vi "VR Example.vi"() -> ()   [LabVIEW 2011]
uses:
  <vilib>/Platform/TimedLoop/XDataNode/timing_clust.ctl
  <vilib>/Platform/TimedLoop/XDataNode/nitl_modes.ctl
  <vilib>/Platform/TimedLoop/XDataNode/wakeup.ctl
  <vilib>/rvi/DataTransferAndStorage/Container/Common/niFpgaContainerState.ctl
  <vilib>/rvi/DataTransferAndStorage/Container/Common/niFpgaDataTypeControl.ctl
  <vilib>/rvi/DataTransferAndStorage/Container/Common/niFpgaContainerImplementationControl.ctl
  <vilib>/rvi/DataTransferAndStorage/Container/Common/niFpgaContainerArbitrationOptionsControl.ctl
  <vilib>/rvi/DataTransferAndStorage/Container/Common/niFpgaTransferTypeControl.ctl
  <vilib>/rvi/DataTransferAndStorage/Container/Common/niFpgaContainerInitializationParameters.ctl
  <vilib>/rvi/Memory/Memory_Types/niFpgaMemoryInterfaceConfiguration.ctl
  <vilib>/rvi/FIFO/Fifo_Types/niFpgaFifoControlLogicControl.ctl
  <vilib>/rvi/DataTransferAndStorage/Container/Common/niFpgaContainerMetaDataKey.ctl
  <userlib>/AES/FPGA/FPGA TypeDefs/aes_FullyCustomTeeth ActionEngine Enum.ctl
  <userlib>/_NI VeriStand FPGA Support/NI VeriStand RIO Library/Custom Device Components/Engine Simulation/Engine Simulation Globals.vi
  <userlib>/AES/FPGA/FPGA VIs/AES ECU Event Measurement - All Measurements.vi
  <vilib>/rvi/DataTransferAndStorage/Container/Common/niFpgaContainerGetUniqueNameForEmu.vi
  <vilib>/rvi/DataTransferAndStorage/Container/Common/niFpgaContainerSetEmuInfo.vi
  <vilib>/rvi/eio/common/nirviEmuReportErrorAndStop.vi
  <vilib>/rvi/Memory/Memory_Emulation/niFpgaMemoryEmulationValidateCache.vi
  <vilib>/rvi/Memory/Memory_Emulation/nirvimemoryEmulationManagerCache_InsertValue.vi
  <vilib>/Utility/error.llb/Clear Errors.vi
  <vilib>/rvi/Memory/Memory_Emulation/nirvimemoryEmulationManagerCache_GetValue.vi
  <vilib>/rvi/Memory/Memory_Emulation/nirvimemoryEmulationManagerCache_SetValue.vi
  <vilib>/rvi/DataTransferAndStorage/Container/Common/niFpgaContainerExecOnDevCompGetState.vi
  <vilib>/rvi/eio/common/nirviEmuTemplateMethod_errors.vi
  <vilib>/rvi/FIFO/Fifo_Resource/nirvififoEmulationSetSize.vi
  <vilib>/Platform/TimedLoop/XDataNode/XDataNode.xnode
  <vilib>/eio/EIONode/EIONode.xnode
  <vilib>/rvi/LocalResourceManager/LocalResourceManager.xnode
  <vilib>/rvi/DataTransferAndStorage/Container/XNode/niFpgaContainer.xnode
  <vilib>/rvi/Memory/Memory_Emulation/nirvimemoryEmulation.vi
  <vilib>/rvi/Memory/Memory_Emulation/niFpgaMemoryEmulationRefIn.vi
  <vilib>/rvi/FIFO/Fifo_Resource/nirvififoEmulationRead.vi
  <vilib>/rvi/FIFO/Fifo_Resource/nirvififoEmulationWrite.vi
  <userlib>/AES/FPGA/AES FPGA.lvlib
  <vilib>/Platform/TimedLoop/XDataNode/XDNodeRunTimeDep.lvlib
panel:
  in  "FullyCustomTeeth.Cams.Cam1.CycleAngle":bool
  in  "DataReplay.Offset.Crankshaft.CKS.1":u64
  in  "DataReplay.ReverseNegate?.Crankshaft.CKS.1":bool
  out "ECUEvent.IC 1.End Angle":u64
  out "ECUEvent.IC 1.Time Duration":u32
  out "ECUEvent.IC 1.Start Angle":u64
  out "ECUEvent.IC 1.Angle Duration":u64
  out "ECUEvent.FI 1.End Angle":u64
  out "ECUEvent.FI 1.Time Duration":u32
  out "ECUEvent.FI 1.Start Angle":u64
  out "ECUEvent.FI 1.Angle Duration":u64
  in  "FullyCustomTeeth.Cams.Cam1.First Rising?":bool
  in  "FullyCustomTeeth.Cams.Num Angles":u8=2
  in  "FullyCustomTeeth.Cams.Cam1.Offset":u64
  in  "FullyCustomTeeth.Cams.Num Profiles":u8=1
  in  "FullyCustomTeeth.Cams.Data":u64
  in  "FullyCustomTeeth.Cams.Toggle":bool
  in  "DataReplay.LoadOffset":u16
  in  "DataReplay.CycleAngle?.Crankshaft.CKS.1":bool
  in  "DataReplay.RPMThreshold.Crankshaft.CKS.1":u64
  in  "DataReplay.VScaleSlope.Crankshaft.CKS.1":u32
  in  "DataReplay.AngleToAddress.Crankshaft.CKS.1":u32
  in  "DataReplay.VScaleIntercept.Crankshaft.CKS.1":i32
  in  "DataReplay.UpdateRate.Crankshaft":u32=400
  in  "APU.Degrees per Tick":u64
  out "APU.Crank Angle":u64
  out "APU.Cycle Angle":u64
  in  "APU.Reset":bool
  in  "APU.Increment Rate":u64
  in  "DataReplay.Data":i16[](array[numeric])=[0, 0, 0, 0, 0, 0, 0, 0, 0, 0, 0, 0, 0, 0, 0, 0, 0, 0, 0, 0, 0, 0, 0, 0, 0, 0, 0, 0, 0, 0, 0, 0]
  in  "DataReplay.LoadDone":bool
  in  "DataReplay.Select":i8
  in  "DataReplay.Toggle":bool
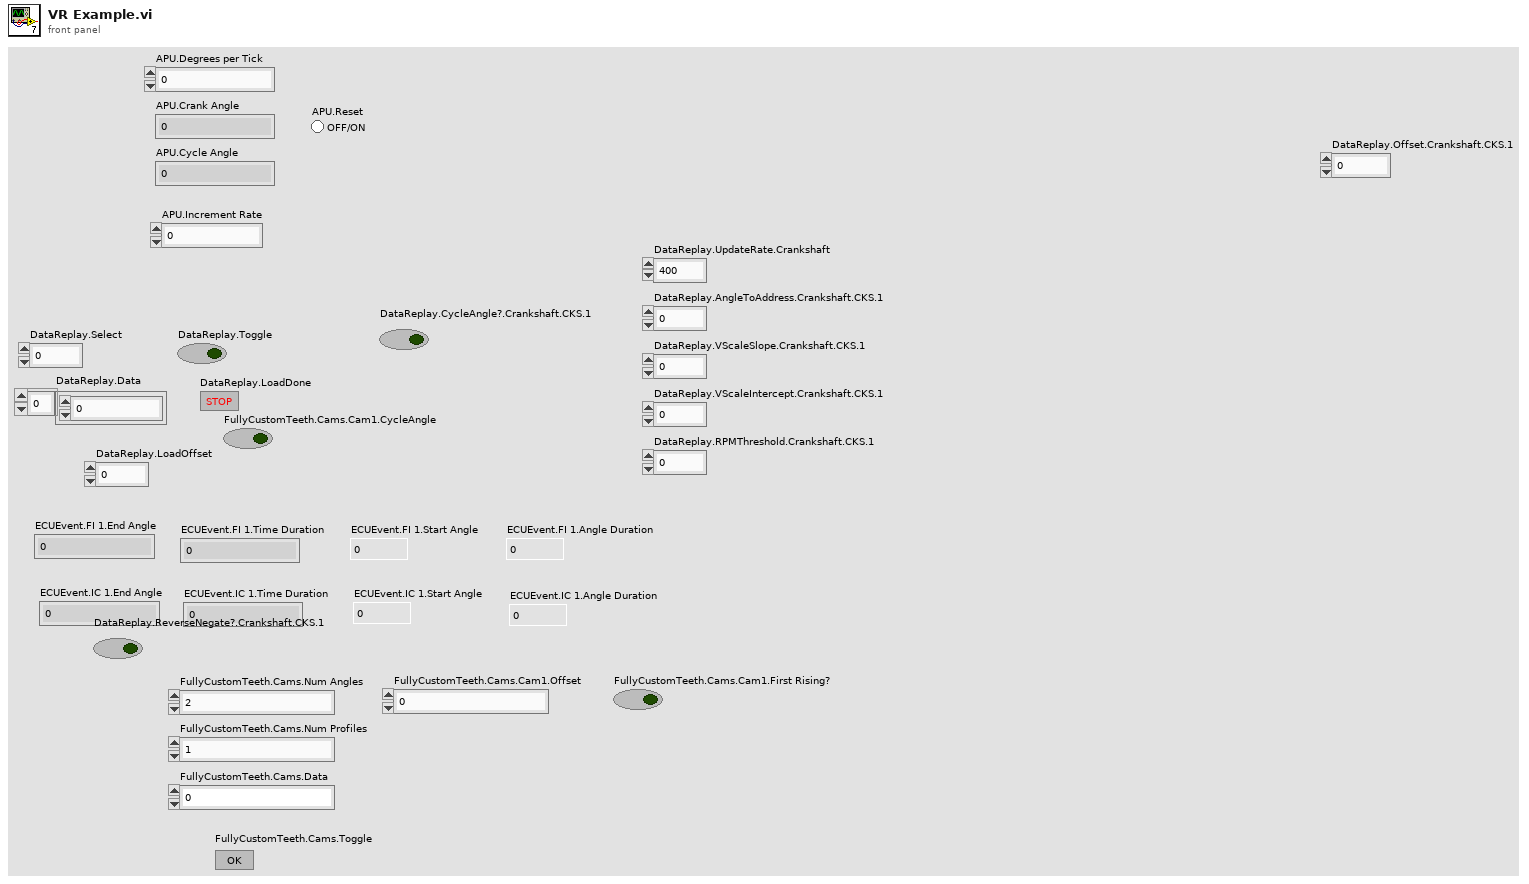
[diagram p1: front panel]
types:
  T1 = typedef "XDNodeRunTimeDep.lvlib/timing_clust.ctl" = cluster{"Expected End [f-1]":u64, "Actual End [f-1]":u64, "Finished Late? [f-1]":bool, "Expected End [i-1]":u64, "Actual End [i-1]":u64, "Finished Late? [i-1]":bool, "Expected Start [i]":u64, "Actual Start [i]":u64, "Expected Start [f]":u64, "Actual Start [f]":u64, "Source Name":string, "Structure Name":string, "Period":i64, "Deadline":i64, "Offset":i64, "Start":i64, "Priority":i32, "Timeout":i32, "Mode":T2, "Wakeup Reason":T3, "Error":errorcluster, "Source Type":string, "Secondary Source Type":string, "Global End Time":u64, "Global Start Time":u64, "Frame Duration":u64, "Iteration Duration":u64, "Assigned CPU":i32, "I/O Scan Engine Mode":u32}
  T2 = typedef "XDNodeRunTimeDep.lvlib/nitl_modes.ctl" = enum32{"No Change", "Process missed periods, maintain original phase", "Discard missed periods, maintain original phase", "Process missed periods, ignore original phase", "Discard missed periods, ignore original phase"}
  T3 = typedef "XDNodeRunTimeDep.lvlib/wakeup.ctl" = enum32{"Normal", "Aborted", "Asynchronous wakeup", "Timing source error", "Timed loop error", "Timeout"}
  T4 = typedef "AES.lvlib/AES FPGA.lvlib/aes_FullyCustomTeeth ActionEngine Enum.ctl" = enum16{"Write Angle", "Update Output"}
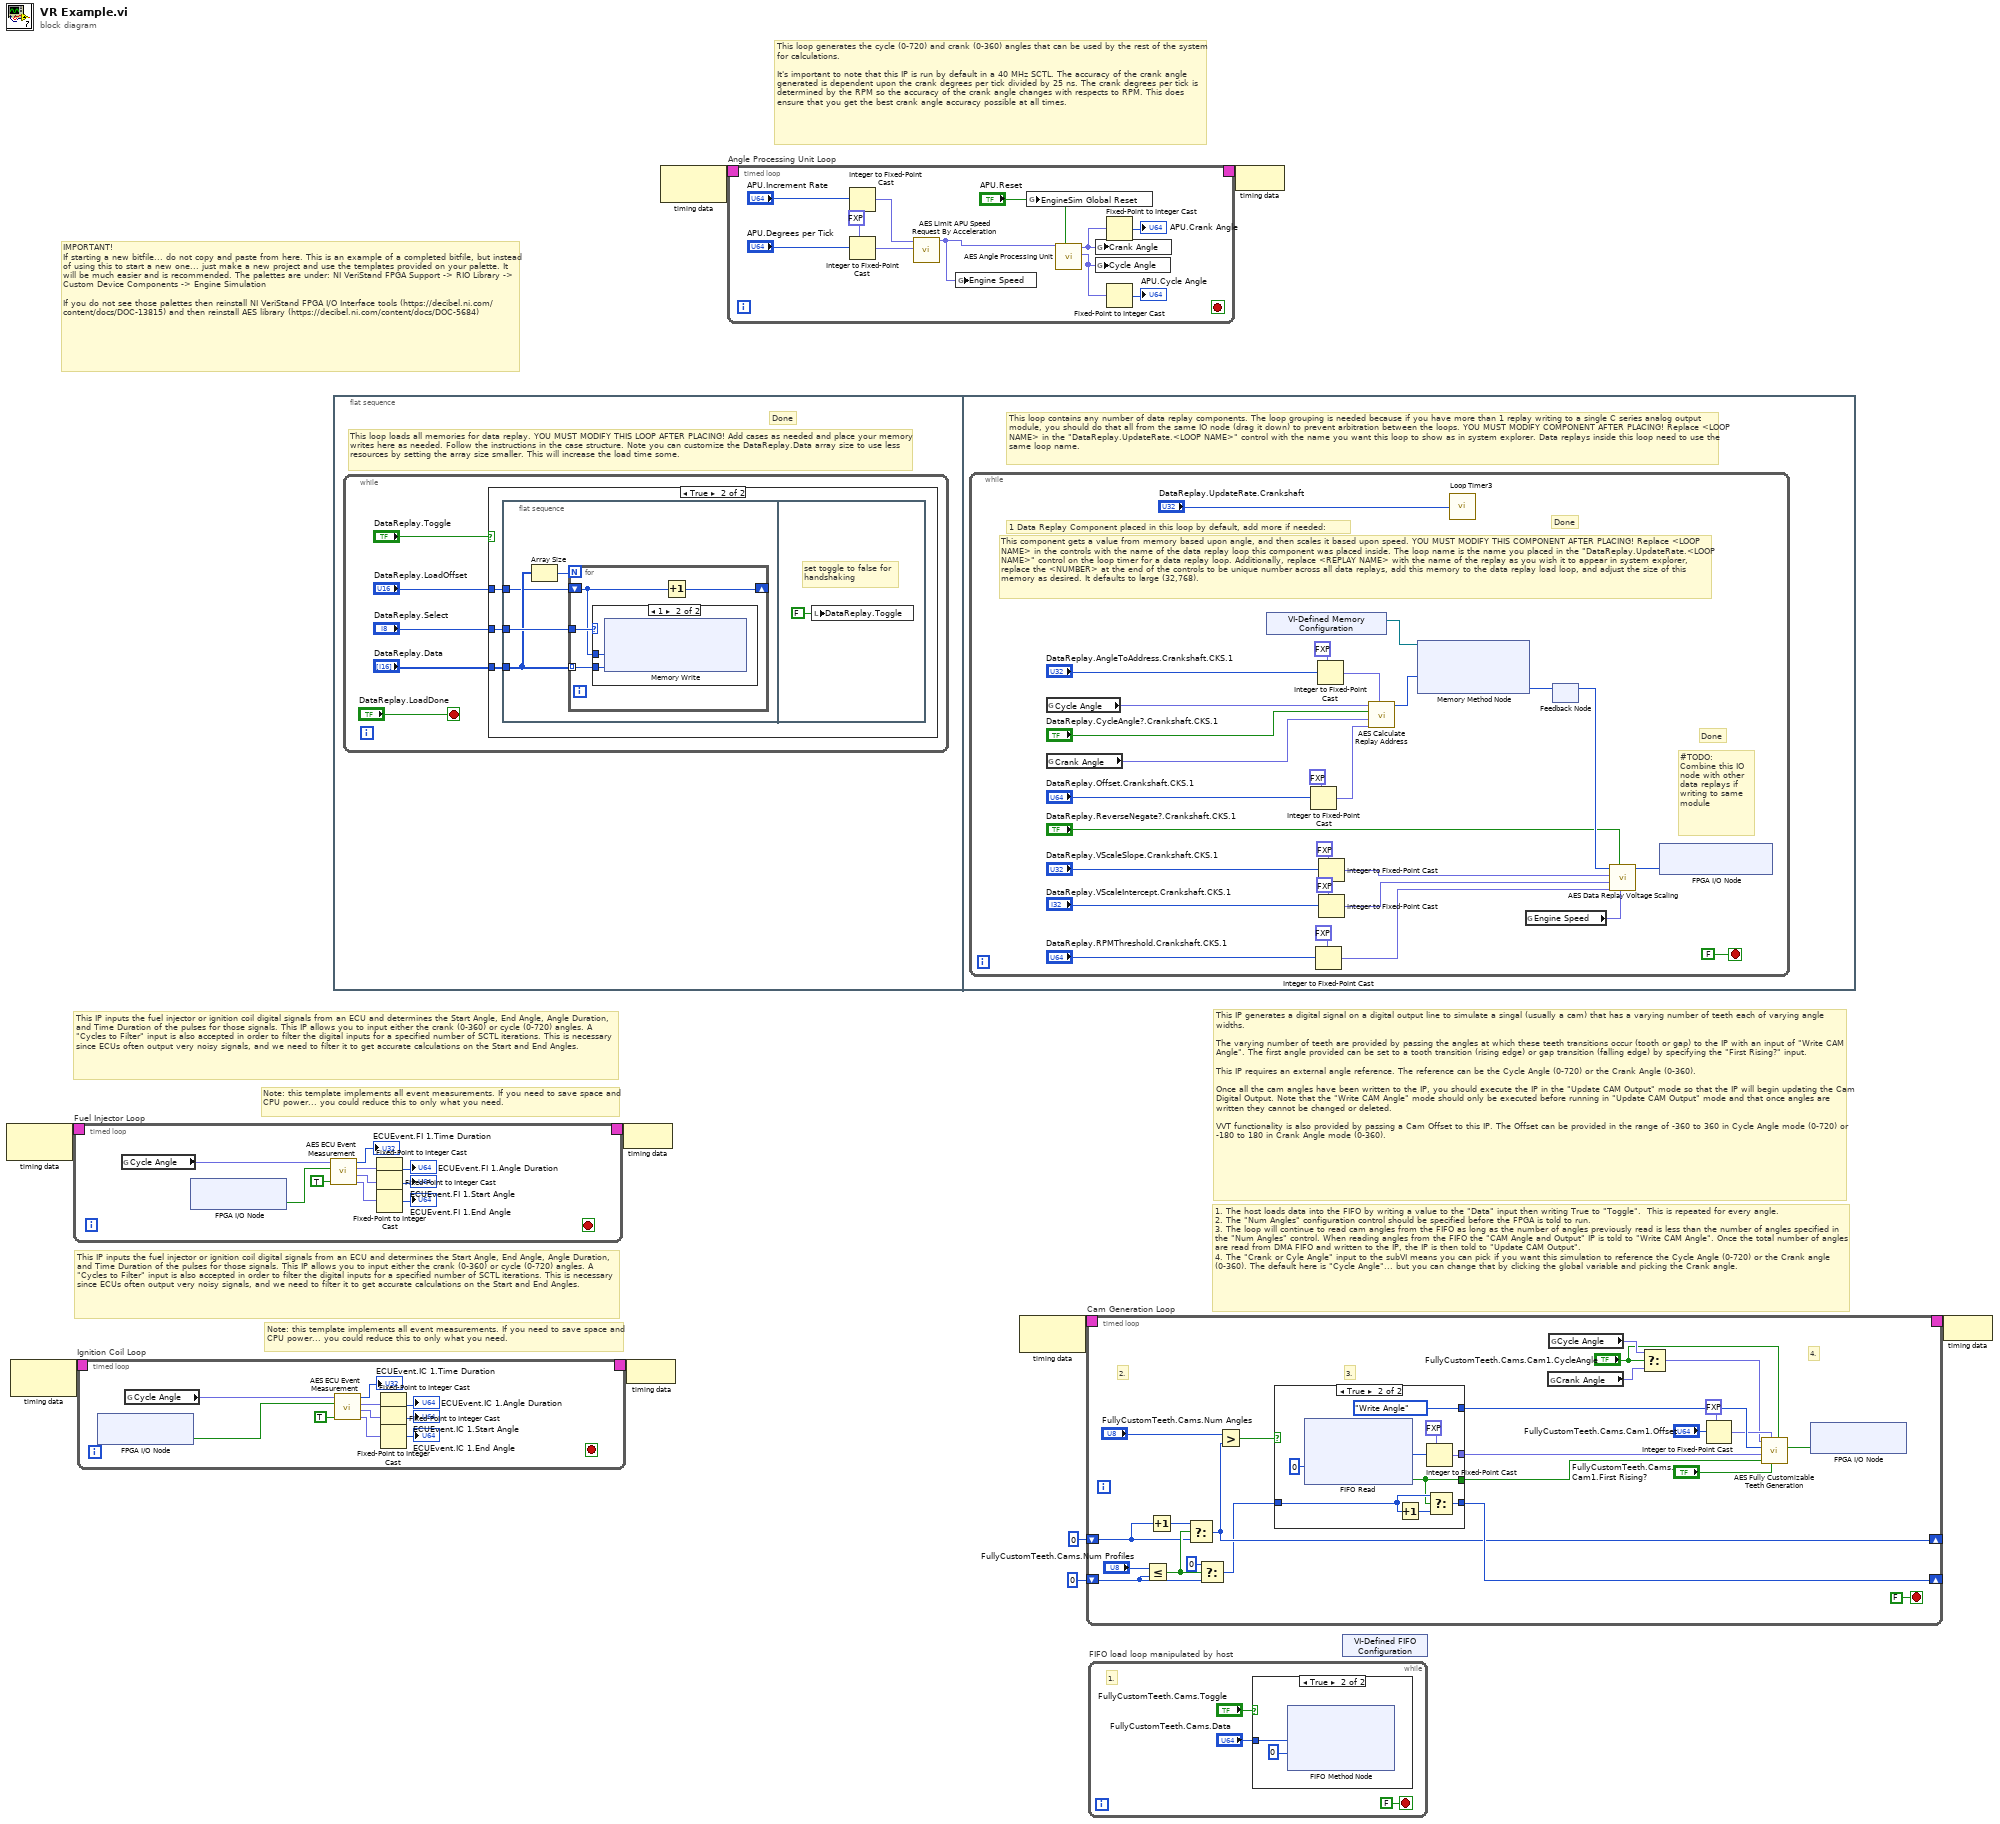
[diagram p0: block diagram]
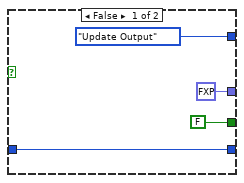
[diagram p3: hidden frame]
diagram:
  # "IMPORTANT!\nIf starting a new bitfile... do not copy and paste from here. This is an example of a completed bitfile, but instead of using this to start a new one... just make a new project and use the templates provided on your palette. It will be much easier and is recommended. The palettes are under: NI VeriStand FPGA Support -> RIO Library -> Custom Device Components -> Engine Simulation\n\nIf you do not see those palettes then reinstall NI VeriStand FPGA I/O Interface tools (https://decibel.ni.com/content/docs/DOC-13815) and then reinstall AES library (https://decibel.ni.com/content/docs/DOC-5684)"
  # "Note: this template implements all event measurements. If you need to save space and CPU power... you could reduce this to only what you need."
  # "This IP inputs the fuel injector or ignition coil digital signals from an ECU and determines the Start Angle, End Angle, Angle Duration, and Time Duration of the pulses for those signals. This IP allows you to input either the crank (0-360) or cycle (0-720) angles. A \"Cycles to Filter\" input is also accepted in order to filter the digital inputs for a specified number of SCTL iterations. This is necessary since ECUs often output very noisy signals, and we need to filter it to get accurate calculations on the Start and End Angles."
  # "Note: this template implements all event measurements. If you need to save space and CPU power... you could reduce this to only what you need."
  # "This IP inputs the fuel injector or ignition coil digital signals from an ECU and determines the Start Angle, End Angle, Angle Duration, and Time Duration of the pulses for those signals. This IP allows you to input either the crank (0-360) or cycle (0-720) angles. A \"Cycles to Filter\" input is also accepted in order to filter the digital inputs for a specified number of SCTL iterations. This is necessary since ECUs often output very noisy signals, and we need to filter it to get accurate calculations on the Start and End Angles."
  # "1. The host loads data into the FIFO by writing a value to the \"Data\" input then writing True to \"Toggle\".  This is repeated for every angle.\n2. The \"Num Angles\" configuration control should be specified before the FPGA is told to run.\n3. The loop will continue to read cam angles from the FIFO as long as the number of angles previously read is less than the number of angles specified in the \"Num Angles\" control. When reading angles from the FIFO the \"CAM Angle and Output\" IP is told to \"Write CAM Angle\". Once the total number of angles are read from DMA FIFO and written to the IP, the IP is then told to \"Update CAM Output\".\n4. The \"Crank or Cyle Angle\" input to the subVI means you can pick if you want this simulation to reference the Cycle Angle (0-720) or the Crank angle (0-360). The default here is \"Cycle Angle\"... but you can change that by clicking the global variable and picking the Crank angle."
  # "This IP generates a digital signal on a digital output line to simulate a singal (usually a cam) that has a varying number of teeth each of varying angle widths. \n\nThe varying number of teeth are provided by passing the angles at which these teeth transitions occur (tooth or gap) to the IP with an input of \"Write CAM Angle\". The first angle provided can be set to a tooth transition (rising edge) or gap transition (falling edge) by specifying the \"First Rising?\" input. \n\nThis IP requires an external angle reference. The reference can be the Cycle Angle (0-720) or the Crank Angle (0-360). \n\nOnce all the cam angles have been written to the IP, you should execute the IP in the \"Update CAM Output\" mode so that the IP will begin updating the Cam Digital Output. Note that the \"Write CAM Angle\" mode should only be executed before running in \"Update CAM Output\" mode and that once angles are written they cannot be changed or deleted.\n\nVVT functionality is also provided by passing a Cam Offset to this IP. The Offset can be provided in the range of -360 to 360 in Cycle Angle mode (0-720) or -180 to 180 in Crank Angle mode (0-360)."
  # "This loop generates the cycle (0-720) and crank (0-360) angles that can be used by the rest of the system for calculations. \n\nIt's important to note that this IP is run by default in a 40 MHz SCTL. The accuracy of the crank angle generated is dependent upon the crank degrees per tick divided by 25 ns. The crank degrees per tick is determined by the RPM so the accuracy of the crank angle changes with respects to RPM. This does ensure that you get the best crank angle accuracy possible at all times."
  n1 = node-c288() -> (w4:T1)  [unwired: 1 out]
  n2 = node-c288() -> (w2:T1)  [unwired: 1 out]
  n3 = timed-loop "Fuel Injector Loop" {
    timing: w4 -> [_]
    timing-out: [_] -> w3
    stop <- _ stop-if-true
    n4 = global read "Engine Simulation Globals.vi" "Cycle Angle"() -> (w20:fxp<+,61,10>)
    n5 = xnode "FPGA I/O Node"() -> ("NI 9401/DIO0"=w12:bool)  [unwired: 1 in, 1 out]
    n6 = call-poly <userlib>:"AES ECU Event Measurement.vi"("Using Cycle Angle"=TRUE, "Digital Input Pulse"=w12, "Crank or Cyle Angle"=w20) -> ("End Angle (degrees)"=w18:fxp<+,61,10>, "Start Angle (degrees)"=w17:fxp<+,61,10>, "Angle Duration (degrees)"=w16:fxp<+/-,62,11>, "Time Duration (clock ticks)"=→"ECUEvent.FI 1.Time Duration":u32)  [unwired: 5 in]
    n7 = Fixed-Point to Integer Cast(1:w16) -> (0:→"ECUEvent.FI 1.Angle Duration":i64)
    n8 = Fixed-Point to Integer Cast(1:w17) -> (0:→"ECUEvent.FI 1.Start Angle":u64)
    n9 = Fixed-Point to Integer Cast(1:w18) -> (0:→"ECUEvent.FI 1.End Angle":u64)
  }
  n10 = timed-loop "Ignition Coil Loop" {
    timing: w2 -> [_]
    timing-out: [_] -> w1
    stop <- _ stop-if-true
    n11 = xnode "FPGA I/O Node"() -> ("NI 9401/DIO1"=w24:bool)  [unwired: 1 in, 1 out]
    n12 = global read "Engine Simulation Globals.vi" "Cycle Angle"() -> (w32:fxp<+,61,10>)
    n13 = call-poly <userlib>:"AES ECU Event Measurement.vi"("Using Cycle Angle"=TRUE, "Digital Input Pulse"=w24, "Crank or Cyle Angle"=w32) -> ("End Angle (degrees)"=w30:fxp<+,61,10>, "Start Angle (degrees)"=w29:fxp<+,61,10>, "Angle Duration (degrees)"=w28:fxp<+/-,62,11>, "Time Duration (clock ticks)"=→"ECUEvent.IC 1.Time Duration":u32)  [unwired: 5 in]
    n14 = Fixed-Point to Integer Cast(1:w28) -> (0:→"ECUEvent.IC 1.Angle Duration":i64)
    n15 = Fixed-Point to Integer Cast(1:w29) -> (0:→"ECUEvent.IC 1.Start Angle":u64)
    n16 = Fixed-Point to Integer Cast(1:w30) -> (0:→"ECUEvent.IC 1.End Angle":u64)
  }
  n17 = flat-sequence {
    frame #0 {
      # "Done"
      # "This loop loads all memories for data replay. YOU MUST MODIFY THIS LOOP AFTER PLACING! Add cases as needed and place your memory writes here as needed. Follow the instructions in the case structure. Note you can customize the DataReplay.Data array size to use less resources by setting the array size smaller. This will increase the load time some."
      n18 = while {
        stop <- "DataReplay.LoadDone" stop-if-true
        n19 = case shown="True" "DataReplay.Toggle" {
          tunnel: "DataReplay.Data" -> [_ w42]
          tunnel: "DataReplay.Select" -> [_ w41]
          tunnel: "DataReplay.LoadOffset" -> [_ w40]
          frame False {
          }
          frame True {
            n20 = flat-sequence {
              tunnel: w42 -> [w45]
              tunnel: w41 -> [w46]
              tunnel: w40 -> [w43]
              frame #0 {
                n21 = Array Size(array=w45) -> (size(s)=w44:i32)
                n22 = for {
                  N: w44 -> [_]
                  tunnel: w45 -> [w48] mode=indexing
                  shift-right: [w50] -> _
                  shift-left: w43 -> [w47]
                  tunnel: w46 -> [w49]
                  n23 = case shown="1" w49 {
                    tunnel: w48 -> [_ w52]
                    tunnel: w47 -> [_ w51]
                    frame Default {
                    }
                    frame 1 {
                      n24 = xnode ("Memory Write")("Address"=w51, "Data"=w52) -> ()  [unwired: 1 in, 1 out]
                    }
                  }
                  n25 = Increment(x=w47) -> (x+1=w50:u16)
                }
              }
              frame #1 {
                # "set toggle to false for\nhandshaking"
                n26 = local write "DataReplay.Toggle"(FALSE ("DataReplay.Toggle")) -> ()
              }
            }
          }
        }
      }
    }
    frame #1 {
      # "This loop contains any number of data replay components. The loop grouping is needed because if you have more than 1 replay writing to a single C series analog output module, you should do that all from the same IO node (drag it down) to prevent arbitration between the loops. YOU MUST MODIFY COMPONENT AFTER PLACING! Replace <LOOP NAME> in the \"DataReplay.UpdateRate.<LOOP NAME>\" control with the name you want this loop to show as in system explorer. Data replays inside this loop need to use the same loop name."
      n27 = while {
        stop <- FALSE stop-if-true
        # "This component gets a value from memory based upon angle, and then scales it based upon speed. YOU MUST MODIFY THIS COMPONENT AFTER PLACING! Replace <LOOP NAME> in the controls with the name of the data replay loop this component was placed inside. The loop name is the name you placed in the \"DataReplay.UpdateRate.<LOOP NAME>\" control on the loop timer for a data replay loop. Additionally, replace <REPLAY NAME> with the name of the replay as you wish it to appear in system explorer, replace the <NUMBER> at the end of the controls to be unique number across all data replays, add this memory to the data replay load loop, and adjust the size of this memory as desired. It defaults to large (32,768)."
        # "Done"
        # "Done"
        # "#TODO:\nCombine this IO node with other data replays if writing to same module"
        # "1 Data Replay Component placed in this loop by default, add more if needed:"
        n28 = global read "Engine Simulation Globals.vi" "Cycle Angle"() -> (w60:fxp<+,61,10>)
        n29 = global read "Engine Simulation Globals.vi" "Crank Angle"() -> (w58:fxp<+,60,9>)
        n30 = xnode "VI-Defined Memory Configuration"() -> ("Memory Out"=w62:refnum<k21>)
        n31 = Integer to Fixed-Point Cast(fixed-point type=fxp<+/-,61,10> 0.0 ("FullyCustomTeeth.Cams.Cam1.Offset"), integer="DataReplay.Offset.Crankshaft.CKS.1") -> (fixed-point=w54:fxp<+/-,61,10>)
        n32 = Integer to Fixed-Point Cast(fixed-point type=fxp<+/-,47,-4> 0.0 ("Crank.Degrees per Tick"), integer="DataReplay.RPMThreshold.Crankshaft.CKS.1") -> (fixed-point=w68:fxp<+/-,47,-4>)
        n33 = Integer to Fixed-Point Cast(fixed-point type=fxp<+,18,7> 0.0 ("Crank.Degrees per Tick"), integer="DataReplay.AngleToAddress.Crankshaft.CKS.1") -> (fixed-point=w61:fxp<+,18,7>)
        n34 = Integer to Fixed-Point Cast(fixed-point type=fxp<+,18,12> 0.0 ("Crank.Degrees per Tick"), integer="DataReplay.VScaleSlope.Crankshaft.CKS.1") -> (fixed-point=w66:fxp<+,18,12>)
        n35 = Integer to Fixed-Point Cast(fixed-point type=fxp<+/-,18,3> 0.0 ("Crank.Degrees per Tick"), integer="DataReplay.VScaleIntercept.Crankshaft.CKS.1") -> (fixed-point=w67:fxp<+/-,18,3>)
        n36 = call <userlib>:"AES Calculate Replay Address.vi"("AngleToAddress"=w61, "Offset (0)"=w54, "Crank Angle"=w58, "CycleAngle?"="DataReplay.CycleAngle?.Crankshaft.CKS.1", "Cycle Angle"=w60) -> ("memory address"=w57:u32)  [unwired: 6 in]
        n37 = xnode ("Memory Method Node")("Address"=w57, "Memory In"=w62) -> ("Data"=w72:i16)  [unwired: 1 out]
        n38 = call "Loop Timer3"("Count(Ticks)"="DataReplay.UpdateRate.Crankshaft") -> ()  [unwired: 1 out]
        n39 = global read "Engine Simulation Globals.vi" "Engine Speed"() -> (w69:fxp<+/-,47,-4>)
        n40 = feedback #1() -> (w65:i16)  [unwired: 1 in]
        n41 = feedback-in #1(w72) -> ()
        n42 = call <userlib>:"AES Data Replay Voltage Scaling.vi"("APU.Degrees per Tick"=w69, "negate voltage when speed negative?"="DataReplay.ReverseNegate?.Crankshaft.CKS.1", "speed threshold"=w68, "voltage scaling intercept"=w67, "voltage scaling slope"=w66, "replay data"=w65) -> ("output value"=w64:i16)  [unwired: 5 in]
        n43 = xnode "FPGA I/O Node"("Connector0/AO0"=w64) -> ()  [unwired: 1 in, 1 out]
      }
    }
  }
  n44 = node-c288(w3) -> ()
  n45 = node-c288(w1) -> ()
  n46 = node-c288() -> (w10:T1)  [unwired: 1 in]
  n47 = timed-loop "Angle Processing Unit Loop" {
    timing: w10 -> [_]
    timing-out: [_] -> w9
    stop <- _ stop-if-true
    w107 = fxp<+/-,47,-4> 0.0 ("Crank.Degrees per Tick")
    n48 = Integer to Fixed-Point Cast(fixed-point type=w107, integer="APU.Increment Rate") -> (fixed-point=w106:fxp<+/-,47,-4>)
    n49 = Integer to Fixed-Point Cast(fixed-point type=w107, integer="APU.Degrees per Tick") -> (fixed-point=w109:fxp<+/-,47,-4>)
    n50 = call <userlib>:"AES Limit APU Speed Request By Acceleration.vi"("APU.Degrees per Tick in"=w109, "APU.Increment Rate"=w106) -> ("APU.Degrees per Tick out"=w105:fxp<+/-,47,-4>)  [unwired: 9 in]
    n51 = global write "Engine Simulation Globals.vi" "Engine Speed"(w105) -> ()
    n52 = global write "Engine Simulation Globals.vi" "EngineSim Global Reset"("APU.Reset") -> ()
    n53 = call <userlib>:"AES Angle Processing Unit.vi"("APU.Reset"="APU.Reset", "APU.Degrees per Tick"=w105) -> ("APU.Cycle Angle"=w111:fxp<+,61,10>, "APU.Crank Angle"=w115:fxp<+,60,9>)  [unwired: 8 in]
    n54 = global write "Engine Simulation Globals.vi" "Crank Angle"(w115) -> ()
    n55 = global write "Engine Simulation Globals.vi" "Cycle Angle"(w111) -> ()
    n56 = Fixed-Point to Integer Cast(1:w115) -> (0:→"APU.Crank Angle":u64)
    n57 = Fixed-Point to Integer Cast(1:w111) -> (0:→"APU.Cycle Angle":u64)
  }
  n58 = node-c288() -> (w8:T1)  [unwired: 1 out]
  n59 = timed-loop "Cam Generation Loop" {
    timing: w8 -> [_]
    timing-out: [_] -> w7
    shift-right: [w139] -> _
    shift-left: u8 0 -> [w132]
    shift-right: [w131] -> _
    shift-left: u8 0 ("CAM.Num Angles") -> [w133]
    stop <- FALSE stop-if-true
    # "4."
    # "3."
    # "2."
    n60 = Less Or Equal?(x="FullyCustomTeeth.Cams.Num Profiles", y=w132) -> (x <= y?=w136:bool)
    n61 = Increment(x=w133) -> (x+1=w135:u8)
    n62 = Select(t=w135, s=w136, f=w133) -> (s? t:f=w131:u8)
    n63 = Select(t=u8 0, s=w136, f=w132) -> (s? t:f=w129:u8)
    n64 = Greater?(x="FullyCustomTeeth.Cams.Num Angles", y=w131) -> (0:w140:bool)
    n65 = case shown="True" w140 {
      tunnel: w129 -> [w145 w152]
      tunnel: [w145 w151] -> w139
      tunnel: [FALSE ("Timed Out?") w150] -> w128
      tunnel: [aes_FullyCustomTeeth_ActionEngine_Enum."Update Output" ("FullyCustomTeeth.Action") aes_FullyCustomTeeth_ActionEngine_Enum."Write Angle" ("FullyCustomTeeth.Action")] -> w126
      tunnel: [fxp<+,61,10> 0.0 ("Element") w147] -> w130
      frame False {
      }
      frame True {
        n66 = xnode ("FIFO Read")("Timeout"=0) -> ("Element"=w149:u64, "Timed Out?"=w150:bool)  [unwired: 1 in, 1 out]
        n67 = Increment(x=w152) -> (x+1=w153:u8)
        n68 = Integer to Fixed-Point Cast(fixed-point type=fxp<+,61,10> 0.0 ("Element"), integer=w149) -> (fixed-point=w147:fxp<+,61,10>)
        n69 = Select(t=w152, s=w150, f=w153) -> (s? t:f=w151:u8)
      }
    }
    n70 = global read "Engine Simulation Globals.vi" "Crank Angle"() -> (w121:fxp<+,60,9>)
    n71 = global read "Engine Simulation Globals.vi" "Cycle Angle"() -> (w120:fxp<+,61,10>)
    n72 = Select(t=w120, s="FullyCustomTeeth.Cams.Cam1.CycleAngle", f=w121) -> (s? t:f=w119:fxp<+,61,10>)
    n73 = Integer to Fixed-Point Cast(fixed-point type=fxp<+/-,61,10> 0.0 ("FullyCustomTeeth.Cams.Cam1.Offset"), integer="FullyCustomTeeth.Cams.Cam1.Offset") -> (fixed-point=w123:fxp<+/-,61,10>)
    n74 = call <userlib>:"AES Fully Customizable Teeth Generation.vi"("Using Cycle Angle"="FullyCustomTeeth.Cams.Cam1.CycleAngle", "FullyCustomTeeth.FirstElement RisingEdge?"="FullyCustomTeeth.Cams.Cam1.First Rising?", "FullyCustomTeeth.Offset"=w123, "Write Timeout?"=w128, "FullyCustomTeeth.Next Angle"=w130, "FullyCustomTeeth.Action"=w126, "Crank or Cyle Angle"=w119) -> ("FullyCustomTeeth.Digital Output"=w127:bool)  [unwired: 4 in]
    n75 = xnode "FPGA I/O Node"("NI 9401/DIO4"=w127) -> ()  [unwired: 1 in, 1 out]
  }
  n76 = while "FIFO load loop manipulated by host" {
    stop <- FALSE stop-if-true
    # "1."
    n77 = case shown="True" "FullyCustomTeeth.Cams.Toggle" {
      tunnel: "FullyCustomTeeth.Cams.Data" -> [_ w161]
      frame False {
      }
      frame True {
        n78 = xnode ("FIFO Method Node")("Element"=w161, "Timeout"=0) -> ()  [unwired: 1 in, 2 out]
      }
    }
  }
  n79 = node-c288(w9) -> ()
  n80 = xnode "VI-Defined FIFO Configuration"() -> ()  [unwired: 1 out]
  n81 = node-c288(w7) -> ()
